vi "GetNextStepsToExecuteJson.vi"(8 "error in (no error)":errorcluster, 10 "beautify JSON?":bool=TRUE, 11 "SequenceManager in":refnum<class "SequenceManager.lvclass">) -> (0 "error out":errorcluster, 1 "Empty Array?":bool, 2 "GetNextStepsToExecuteAsJson":string, 3 "SequenceManager out":refnum<class "SequenceManager.lvclass">)   [LabVIEW 2023, in "Easy.SequenceManagerLabVIEW.lvlib" / "SequenceManager.lvclass"]
uses:
  SequenceManager.lvclass
  SequenceManager.lvclass/SequenceManager.ctl
  C:/Projects/Cutiss/SequenceManager/SequenceManager/LabViewWrapper/build/Easy.SequenceManager.dll
  build/Easy.SequenceManager.dll
panel:
  # "Connector Pane"
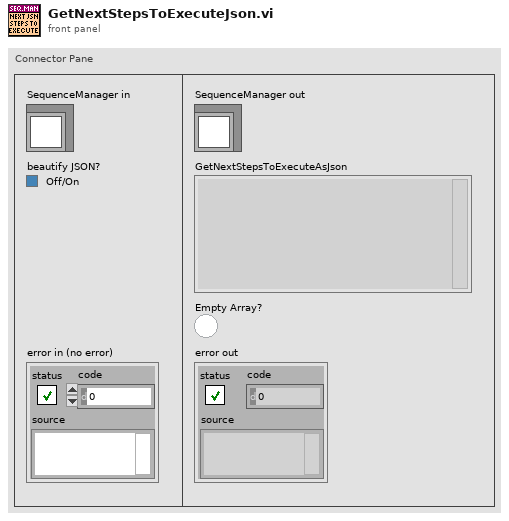
[diagram p1: front panel]
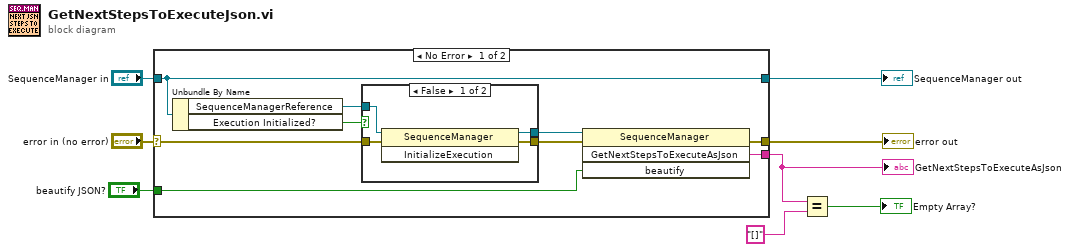
[diagram p0: block diagram]
diagram:
  n1 = case shown="No Error" "error in (no error)" {
    selector: "error in (no error)" -> [w14 w25]
    tunnel: [w11 w25] -> w7
    tunnel: [w17 w24] -> w5
    tunnel: "SequenceManager in" -> [w17 w24]
    tunnel: [w10 _] -> w3
    tunnel: "beautify JSON?" -> [w9 _]
    frame No Error {
      n2 = Unbundle By Name(w17) -> ("SequenceManagerReference"=w15:refnum<k24>, "Execution Initialized?"=w16:bool)
      n3 = case shown="False" w16 {
        tunnel: w15 -> [w20 w23]
        tunnel: [w19 w23] -> w13
        tunnel: w14 -> [w21 w22]
        tunnel: [w18 w22] -> w12
        frame False {
          n4 = invoke class="SequenceManager" method="InitializeExecution"(reference=w20, error in=w21) -> (reference out=w19:refnum<k24>, error out=w18:errorcluster)  [unwired: 1 in, 1 out]
        }
        frame True {
        }
      }
      n5 = invoke class="SequenceManager" method="GetNextStepsToExecuteAsJson"(reference=w13, error in=w12, "beautify"=w9) -> (error out=w11:errorcluster, "GetNextStepsToExecuteAsJson"=w10:string)  [unwired: 1 in, 2 out]
    }
    frame Error {
    }
  }
  "error out" <- w7
  "SequenceManager out" <- w5
  "GetNextStepsToExecuteAsJson" <- w3
  n6 = Equal?(x=w3, y="[]") -> (x = y?=→"Empty Array?":bool)
